vi "FipsAdjacent.vi"() -> (11 "Fips":i32[](array[numeric]))   [LabVIEW 2017] (continued)
\"Deuel County, NE\"\t31049\t\"Keith County, NE\"\t31101\n\"Deuel County, NE\"\t31049\t\"Perkins County, NE\"\t31135\n\"Dixon County, NE\"\t31051\t\"Cedar County, NE\"\t31027\n\"Dixon County, NE\"\t31051\t\"Dakota County, NE\"\t31043\n\"Dixon County, NE\"\t31051\t\"Dixon County, NE\"\t31051\n\"Dixon County, NE\"\t31051\t\"Thurston County, NE\"\t31173\n\"Dixon County, NE\"\t31051\t\"Wayne County, NE\"\t31179\n\"Dixon County, NE\"\t31051\t\"Clay County, SD\"\t46027\n\"Dixon County, NE\"\t31051\t\"Union County, SD\"\t46127\n\"Dodge County, NE\"\t31053\t\"Burt County, NE\"\t31021\n\"Dodge County, NE\"\t31053\t\"Butler County, NE\"\t31023\n\"Dodge County, NE\"\t31053\t\"Colfax County, NE\"\t31037\n\"Dodge County, NE\"\t31053\t\"Cuming County, NE\"\t31039\n\"Dodge County, NE\"\t31053\t\"Dodge County, NE\"\t31053\n\"Dodge County, NE\"\t31053\t\"Douglas County, NE\"\t31055\n\"Dodge County, NE\"\t31053\t\"Saunders County, NE\"\t31155\n\"Dodge County, NE\"\t31053\t\"Washington County, NE\"\t31177\n\"Douglas County, NE\"\t31055\t\"Pottawattamie County, IA\"\t19155\n\"Douglas County, NE\"\t31055\t\"Dodge County, NE\"\t31053\n\"Douglas County, NE\"\t31055\t\"Douglas County, NE\"\t31055\n\"Douglas County, NE\"\t31055\t\"Sarpy County, NE\"\t31153\n\"Douglas County, NE\"\t31055\t\"Saunders County, NE\"\t31155\n\"Douglas County, NE\"\t31055\t\"Washington County, NE\"\t31177\n\"Dundy County, NE\"\t31057\t\"Yuma County, CO\"\t08125\n\"Dundy County, NE\"\t31057\t\"Cheyenne County, KS\"\t20023\n\"Dundy County, NE\"\t31057\t\"Rawlins County, KS\"\t20153\n\"Dundy County, NE\"\t31057\t\"Chase County, NE\"\t31029\n\"Dundy County, NE\"\t31057\t\"Dundy County, NE\"\t31057\n\"Dundy County, NE\"\t31057\t\"Hayes County, NE\"\t31085\n\"Dundy County, NE\"\t31057\t\"Hitchcock County, NE\"\t31087\n\"Fillmore County, NE\"\t31059\t\"Clay County, NE\"\t31035\n\"Fillmore County, NE\"\t31059\t\"Fillmore County, NE\"\t31059\n\"Fillmore County, NE\"\t31059\t\"Jefferson County, NE\"\t31095\n\"Fillmore County, NE\"\t31059\t\"Nuckolls County, NE\"\t31129\n\"Fillmore County, NE\"\t31059\t\"Saline County, NE\"\t31151\n\"Fillmore County, NE\"\t31059\t\"Seward County, NE\"\t31159\n\"Fillmore County, NE\"\t31059\t\"Thayer County, NE\"\t31169\n\"Fillmore County, NE\"\t31059\t\"York County, NE\"\t31185\n\"Franklin County, NE\"\t31061\t\"Phillips County, KS\"\t20147\n\"Franklin County, NE\"\t31061\t\"Smith County, KS\"\t20183\n\"Franklin County, NE\"\t31061\t\"Franklin County, NE\"\t31061\n\"Franklin County, NE\"\t31061\t\"Harlan County, NE\"\t31083\n\"Franklin County, NE\"\t31061\t\"Kearney County, NE\"\t31099\n\"Franklin County, NE\"\t31061\t\"Phelps County, NE\"\t31137\n\"Franklin County, NE\"\t31061\t\"Webster County, NE\"\t31181\n\"Frontier County, NE\"\t31063\t\"Dawson County, NE\"\t31047\n\"Frontier County, NE\"\t31063\t\"Frontier County, NE\"\t31063\n\"Frontier County, NE\"\t31063\t\"Furnas County, NE\"\t31065\n\"Frontier County, NE\"\t31063\t\"Gosper County, NE\"\t31073\n\"Frontier County, NE\"\t31063\t\"Hayes County, NE\"\t31085\n\"Frontier County, NE\"\t31063\t\"Hitchcock County, NE\"\t31087\n\"Frontier County, NE\"\t31063\t\"Lincoln County, NE\"\t31111\n\"Frontier County, NE\"\t31063\t\"Red Willow County, NE\"\t31145\n\"Furnas County, NE\"\t31065\t\"Decatur County, KS\"\t20039\n\"Furnas County, NE\"\t31065\t\"Norton County, KS\"\t20137\n\"Furnas County, NE\"\t31065\t\"Frontier County, NE\"\t31063\n\"Furnas County, NE\"\t31065\t\"Furnas County, NE\"\t31065\n\"Furnas County, NE\"\t31065\t\"Gosper County, NE\"\t31073\n\"Furnas County, NE\"\t31065\t\"Harlan County, NE\"\t31083\n\"Furnas County, NE\"\t31065\t\"Phelps County, NE\"\t31137\n\"Furnas County, NE\"\t31065\t\"Red Willow County, NE\"\t31145\n\"Gage County, NE\"\t31067\t\"Marshall County, KS\"\t20117\n\"Gage County, NE\"\t31067\t\"Washington County, KS\"\t20201\n\"Gage County, NE\"\t31067\t\"Gage County, NE\"\t31067\n\"Gage County, NE\"\t31067\t\"Jefferson County, NE\"\t31095\n\"Gage County, NE\"\t31067\t\"Johnson County, NE\"\t31097\n\"Gage County, NE\"\t31067\t\"Lancaster County, NE\"\t31109\n\"Gage County, NE\"\t31067\t\"Otoe County, NE\"\t31131\n\"Gage County, NE\"\t31067\t\"Pawnee County, NE\"\t31133\n\"Gage County, NE\"\t31067\t\"Saline County, NE\"\t31151\n\"Garden County, NE\"\t31069\t\"Arthur County, NE\"\t31005\n\"Garden County, NE\"\t31069\t\"Cheyenne County, NE\"\t31033\n\"Garden County, NE\"\t31069\t\"Deuel County, NE\"\t31049\n\"Garden County, NE\"\t31069\t\"Garden County, NE\"\t31069\n\"Garden County, NE\"\t31069\t\"Grant County, NE\"\t31075\n\"Garden County, NE\"\t31069\t\"Keith County, NE\"\t31101\n\"Garden County, NE\"\t31069\t\"Morrill County, NE\"\t31123\n\"Garden County, NE\"\t31069\t\"Sheridan County, NE\"\t31161\n\"Garfield County, NE\"\t31071\t\"Custer County, NE\"\t31041\n\"Garfield County, NE\"\t31071\t\"Garfield County, NE\"\t31071\n\"Garfield County, NE\"\t31071\t\"Holt County, NE\"\t31089\n\"Garfield County, NE\"\t31071\t\"Loup County, NE\"\t31115\n\"Garfield County, NE\"\t31071\t\"Valley County, NE\"\t31175\n\"Garfield County, NE\"\t31071\t\"Wheeler County, NE\"\t31183\n\"Gosper County, NE\"\t31073\t\"Dawson County, NE\"\t31047\n\"Gosper County, NE\"\t31073\t\"Frontier County, NE\"\t31063\n\"Gosper County, NE\"\t31073\t\"Furnas County, NE\"\t31065\n\"Gosper County, NE\"\t31073\t\"Gosper County, NE\"\t31073\n\"Gosper County, NE\"\t31073\t\"Phelps County, NE\"\t31137\n\"Grant County, NE\"\t31075\t\"Arthur County, NE\"\t31005\n\"Grant County, NE\"\t31075\t\"Cherry County, NE\"\t31031\n\"Grant County, NE\"\t31075\t\"Garden County, NE\"\t31069\n\"Grant County, NE\"\t31075\t\"Grant County, NE\"\t31075\n\"Grant County, NE\"\t31075\t\"Hooker County, NE\"\t31091\n\"Grant County, NE\"\t31075\t\"Sheridan County, NE\"\t31161\n\"Greeley County, NE\"\t31077\t\"Boone County, NE\"\t31011\n\"Greeley County, NE\"\t31077\t\"Greeley County, NE\"\t31077\n\"Greeley County, NE\"\t31077\t\"Howard County, NE\"\t31093\n\"Greeley County, NE\"\t31077\t\"Nance County, NE\"\t31125\n\"Greeley County, NE\"\t31077\t\"Sherman County, NE\"\t31163\n\"Greeley County, NE\"\t31077\t\"Valley County, NE\"\t31175\n\"Greeley County, NE\"\t31077\t\"Wheeler County, NE\"\t31183\n\"Hall County, NE\"\t31079\t\"Adams County, NE\"\t31001\n\"Hall County, NE\"\t31079\t\"Buffalo County, NE\"\t31019\n\"Hall County, NE\"\t31079\t\"Hall County, NE\"\t31079\n\"Hall County, NE\"\t31079\t\"Hamilton County, NE\"\t31081\n\"Hall County, NE\"\t31079\t\"Howard County, NE\"\t31093\n\"Hall County, NE\"\t31079\t\"Merrick County, NE\"\t31121\n\"Hamilton County, NE\"\t31081\t\"Adams County, NE\"\t31001\n\"Hamilton County, NE\"\t31081\t\"Clay County, NE\"\t31035\n\"Hamilton County, NE\"\t31081\t\"Hall County, NE\"\t31079\n\"Hamilton County, NE\"\t31081\t\"Hamilton County, NE\"\t31081\n\"Hamilton County, NE\"\t31081\t\"Merrick County, NE\"\t31121\n\"Hamilton County, NE\"\t31081\t\"Polk County, NE\"\t31143\n\"Hamilton County, NE\"\t31081\t\"York County, NE\"\t31185\n\"Harlan County, NE\"\t31083\t\"Norton County, KS\"\t20137\n\"Harlan County, NE\"\t31083\t\"Phillips County, KS\"\t20147\n\"Harlan County, NE\"\t31083\t\"Franklin County, NE\"\t31061\n\"Harlan County, NE\"\t31083\t\"Furnas County, NE\"\t31065\n\"Harlan County, NE\"\t31083\t\"Harlan County, NE\"\t31083\n\"Harlan County, NE\"\t31083\t\"Kearney County, NE\"\t31099\n\"Harlan County, NE\"\t31083\t\"Phelps County, NE\"\t31137\n\"Hayes County, NE\"\t31085\t\"Chase County, NE\"\t31029\n\"Hayes County, NE\"\t31085\t\"Dundy County, NE\"\t31057\n\"Hayes County, NE\"\t31085\t\"Frontier County, NE\"\t31063\n\"Hayes County, NE\"\t31085\t\"Hayes County, NE\"\t31085\n\"Hayes County, NE\"\t31085\t\"Hitchcock County, NE\"\t31087\n\"Hayes County, NE\"\t31085\t\"Lincoln County, NE\"\t31111\n\"Hayes County, NE\"\t31085\t\"Perkins County, NE\"\t31135\n\"Hitchcock County, NE\"\t31087\t\"Rawlins County, KS\"\t20153\n\"Hitchcock County, NE\"\t31087\t\"Dundy County, NE\"\t31057\n\"Hitchcock County, NE\"\t31087\t\"Frontier County, NE\"\t31063\n\"Hitchcock County, NE\"\t31087\t\"Hayes County, NE\"\t31085\n\"Hitchcock County, NE\"\t31087\t\"Hitchcock County, NE\"\t31087\n\"Hitchcock County, NE\"\t31087\t\"Red Willow County, NE\"\t31145\n\"Holt County, NE\"\t31089\t\"Antelope County, NE\"\t31003\n\"Holt County, NE\"\t31089\t\"Boyd County, NE\"\t31015\n\"Holt County, NE\"\t31089\t\"Garfield County, NE\"\t31071\n\"Holt County, NE\"\t31089\t\"Holt County, NE\"\t31089\n\"Holt County, NE\"\t31089\t\"Keya Paha County, NE\"\t31103\n\"Holt County, NE\"\t31089\t\"Knox County, NE\"\t31107\n\"Holt County, NE\"\t31089\t\"Loup County, NE\"\t31115\n\"Holt County, NE\"\t31089\t\"Rock County, NE\"\t31149\n\"Holt County, NE\"\t31089\t\"Wheeler County, NE\"\t31183\n\"Hooker County, NE\"\t31091\t\"Arthur County, NE\"\t31005\n\"Hooker County, NE\"\t31091\t\"Cherry County, NE\"\t31031\n\"Hooker County, NE\"\t31091\t\"Grant County, NE\"\t31075\n\"Hooker County, NE\"\t31091\t\"Hooker County, NE\"\t31091\n\"Hooker County, NE\"\t31091\t\"McPherson County, NE\"\t31117\n\"Hooker County, NE\"\t31091\t\"Thomas County, NE\"\t31171\n\"Howard County, NE\"\t31093\t\"Buffalo County, NE\"\t31019\n\"Howard County, NE\"\t31093\t\"Greeley County, NE\"\t31077\n\"Howard County, NE\"\t31093\t\"Hall County, NE\"\t31079\n\"Howard County, NE\"\t31093\t\"Howard County, NE\"\t31093\n\"Howard County, NE\"\t31093\t\"Merrick County, NE\"\t31121\n\"Howard County, NE\"\t31093\t\"Nance County, NE\"\t31125\n\"Howard County, NE\"\t31093\t\"Sherman County, NE\"\t31163\n\"Jefferson County, NE\"\t31095\t\"Republic County, KS\"\t20157\n\"Jefferson County, NE\"\t31095\t\"Washington County, KS\"\t20201\n\"Jefferson County, NE\"\t31095\t\"Fillmore County, NE\"\t31059\n\"Jefferson County, NE\"\t31095\t\"Gage County, NE\"\t31067\n\"Jefferson County, NE\"\t31095\t\"Jefferson County, NE\"\t31095\n\"Jefferson County, NE\"\t31095\t\"Saline County, NE\"\t31151\n\"Jefferson County, NE\"\t31095\t\"Thayer County, NE\"\t31169\n\"Johnson County, NE\"\t31097\t\"Gage County, NE\"\t31067\n\"Johnson County, NE\"\t31097\t\"Johnson County, NE\"\t31097\n\"Johnson County, NE\"\t31097\t\"Lancaster County, NE\"\t31109\n\"Johnson County, NE\"\t31097\t\"Nemaha County, NE\"\t31127\n\"Johnson County, NE\"\t31097\t\"Otoe County, NE\"\t31131\n\"Johnson County, NE\"\t31097\t\"Pawnee County, NE\"\t31133\n\"Kearney County, NE\"\t31099\t\"Adams County, NE\"\t31001\n\"Kearney County, NE\"\t31099\t\"Buffalo County, NE\"\t31019\n\"Kearney County, NE\"\t31099\t\"Franklin County, NE\"\t31061\n\"Kearney County, NE\"\t31099\t\"Harlan County, NE\"\t31083\n\"Kearney County, NE\"\t31099\t\"Kearney County, NE\"\t31099\n\"Kearney County, NE\"\t31099\t\"Phelps County, NE\"\t31137\n\"Kearney County, NE\"\t31099\t\"Webster County, NE\"\t31181\n\"Keith County, NE\"\t31101\t\"Arthur County, NE\"\t31005\n\"Keith County, NE\"\t31101\t\"Deuel County, NE\"\t31049\n\"Keith County, NE\"\t31101\t\"Garden County, NE\"\t31069\n\"Keith County, NE\"\t31101\t\"Keith County, NE\"\t31101\n\"Keith County, NE\"\t31101\t\"Lincoln County, NE\"\t31111\n\"Keith County, NE\"\t31101\t\"McPherson County, NE\"\t31117\n\"Keith County, NE\"\t31101\t\"Perkins County, NE\"\t31135\n\"Keya Paha County, NE\"\t31103\t\"Boyd County, NE\"\t31015\n\"Keya Paha County, NE\"\t31103\t\"Brown County, NE\"\t31017\n\"Keya Paha County, NE\"\t31103\t\"Cherry County, NE\"\t31031\n\"Keya Paha County, NE\"\t31103\t\"Holt County, NE\"\t31089\n\"Keya Paha County, NE\"\t31103\t\"Keya Paha County, NE\"\t31103\n\"Keya Paha County, NE\"\t31103\t\"Rock County, NE\"\t31149\n\"Keya Paha County, NE\"\t31103\t\"Gregory County, SD\"\t46053\n\"Keya Paha County, NE\"\t31103\t\"Todd County, SD\"\t46121\n\"Keya Paha County, NE\"\t31103\t\"Tripp County, SD\"\t46123\n\"Kimball County, NE\"\t31105\t\"Logan County, CO\"\t08075\n\"Kimball County, NE\"\t31105\t\"Weld County, CO\"\t08123\n\"Kimball County, NE\"\t31105\t\"Banner County, NE\"\t31007\n\"Kimball County, NE\"\t31105\t\"Cheyenne County, NE\"\t31033\n\"Kimball County, NE\"\t31105\t\"Kimball County, NE\"\t31105\n\"Kimball County, NE\"\t31105\t\"Laramie County, WY\"\t56021\n\"Knox County, NE\"\t31107\t\"Antelope County, NE\"\t31003\n\"Knox County, NE\"\t31107\t\"Boyd County, NE\"\t31015\n\"Knox County, NE\"\t31107\t\"Cedar County, NE\"\t31027\n\"Knox County, NE\"\t31107\t\"Holt County, NE\"\t31089\n\"Knox County, NE\"\t31107\t\"Knox County, NE\"\t31107\n\"Knox County, NE\"\t31107\t\"Pierce County, NE\"\t31139\n\"Knox County, NE\"\t31107\t\"Bon Homme County, SD\"\t46009\n\"Knox County, NE\"\t31107\t\"Charles Mix County, SD\"\t46023\n\"Knox County, NE\"\t31107\t\"Yankton County, SD\"\t46135\n\"Lancaster County, NE\"\t31109\t\"Butler County, NE\"\t31023\n\"Lancaster County, NE\"\t31109\t\"Cass County, NE\"\t31025\n\"Lancaster County, NE\"\t31109\t\"Gage County, NE\"\t31067\n\"Lancaster County, NE\"\t31109\t\"Johnson County, NE\"\t31097\n\"Lancaster County, NE\"\t31109\t\"Lancaster County, NE\"\t31109\n\"Lancaster County, NE\"\t31109\t\"Otoe County, NE\"\t31131\n\"Lancaster County, NE\"\t31109\t\"Saline County, NE\"\t31151\n\"Lancaster County, NE\"\t31109\t\"Saunders County, NE\"\t31155\n\"Lancaster County, NE\"\t31109\t\"Seward County, NE\"\t31159\n\"Lincoln County, NE\"\t31111\t\"Custer County, NE\"\t31041\n\"Lincoln County, NE\"\t31111\t\"Dawson County, NE\"\t31047\n\"Lincoln County, NE\"\t31111\t\"Frontier County, NE\"\t31063\n\"Lincoln County, NE\"\t31111\t\"Hayes County, NE\"\t31085\n\"Lincoln County, NE\"\t31111\t\"Keith County, NE\"\t31101\n\"Lincoln County, NE\"\t31111\t\"Lincoln County, NE\"\t31111\n\"Lincoln County, NE\"\t31111\t\"Logan County, NE\"\t31113\n\"Lincoln County, NE\"\t31111\t\"McPherson County, NE\"\t31117\n\"Lincoln County, NE\"\t31111\t\"Perkins County, NE\"\t31135\n\"Logan County, NE\"\t31113\t\"Blaine County, NE\"\t31009\n\"Logan County, NE\"\t31113\t\"Custer County, NE\"\t31041\n\"Logan County, NE\"\t31113\t\"Lincoln County, NE\"\t31111\n\"Logan County, NE\"\t31113\t\"Logan County, NE\"\t31113\n\"Logan County, NE\"\t31113\t\"McPherson County, NE\"\t31117\n\"Logan County, NE\"\t31113\t\"Thomas County, NE\"\t31171\n\"Loup County, NE\"\t31115\t\"Blaine County, NE\"\t31009\n\"Loup County, NE\"\t31115\t\"Brown County, NE\"\t31017\n\"Loup County, NE\"\t31115\t\"Custer County, NE\"\t31041\n\"Loup County, NE\"\t31115\t\"Garfield County, NE\"\t31071\n\"Loup County, NE\"\t31115\t\"Holt County, NE\"\t31089\n\"Loup County, NE\"\t31115\t\"Loup County, NE\"\t31115\n\"Loup County, NE\"\t31115\t\"Rock County, NE\"\t31149\n\"McPherson County, NE\"\t31117\t\"Arthur County, NE\"\t31005\n\"McPherson County, NE\"\t31117\t\"Hooker County, NE\"\t31091\n\"McPherson County, NE\"\t31117\t\"Keith County, NE\"\t31101\n\"McPherson County, NE\"\t31117\t\"Lincoln County, NE\"\t31111\n\"McPherson County, NE\"\t31117\t\"Logan County, NE\"\t31113\n\"McPherson County, NE\"\t31117\t\"McPherson County, NE\"\t31117\n\"McPherson County, NE\"\t31117\t\"Thomas County, NE\"\t31171\n\"Madison County, NE\"\t31119\t\"Antelope County, NE\"\t31003\n\"Madison County, NE\"\t31119\t\"Boone County, NE\"\t31011\n\"Madison County, NE\"\t31119\t\"Madison County, NE\"\t31119\n\"Madison County, NE\"\t31119\t\"Pierce County, NE\"\t31139\n\"Madison County, NE\"\t31119\t\"Platte County, NE\"\t31141\n\"Madison County, NE\"\t31119\t\"Stanton County, NE\"\t31167\n\"Madison County, NE\"\t31119\t\"Wayne County, NE\"\t31179\n\"Merrick County, NE\"\t31121\t\"Hall County, NE\"\t31079\n\"Merrick County, NE\"\t31121\t\"Hamilton County, NE\"\t31081\n\"Merrick County, NE\"\t31121\t\"Howard County, NE\"\t31093\n\"Merrick County, NE\"\t31121\t\"Merrick County, NE\"\t31121\n\"Merrick County, NE\"\t31121\t\"Nance County, NE\"\t31125\n\"Merrick County, NE\"\t31121\t\"Platte County, NE\"\t31141\n\"Merrick County, NE\"\t31121\t\"Polk County, NE\"\t31143\n\"Morrill County, NE\"\t31123\t\"Banner County, NE\"\t31007\n\"Morrill County, NE\"\t31123\t\"Box Butte County, NE\"\t31013\n\"Morrill County, NE\"\t31123\t\"Cheyenne County, NE\"\t31033\n\"Morrill County, NE\"\t31123\t\"Garden County, NE\"\t31069\n\"Morrill County, NE\"\t31123\t\"Morrill County, NE\"\t31123\n\"Morrill County, NE\"\t31123\t\"Scotts Bluff County, NE\"\t31157\n\"Morrill County, NE\"\t31123\t\"Sheridan County, NE\"\t31161\n\"Nance County, NE\"\t31125\t\"Boone County, NE\"\t31011\n\"Nance County, NE\"\t31125\t\"Greeley County, NE\"\t31077\n\"Nance County, NE\"\t31125\t\"Howard County, NE\"\t31093\n\"Nance County, NE\"\t31125\t\"Merrick County, NE\"\t31121\n\"Nance County, NE\"\t31125\t\"Nance County, NE\"\t31125\n\"Nance County, NE\"\t31125\t\"Platte County, NE\"\t31141\n\"Nemaha County, NE\"\t31127\t\"Atchison County, MO\"\t29005\n\"Nemaha County, NE\"\t31127\t\"Holt County, MO\"\t29087\n\"Nemaha County, NE\"\t31127\t\"Johnson County, NE\"\t31097\n\"Nemaha County, NE\"\t31127\t\"Nemaha County, NE\"\t31127\n\"Nemaha County, NE\"\t31127\t\"Otoe County, NE\"\t31131\n\"Nemaha County, NE\"\t31127\t\"Pawnee County, NE\"\t31133\n\"Nemaha County, NE\"\t31127\t\"Richardson County, NE\"\t31147\n\"Nuckolls County, NE\"\t31129\t\"Jewell County, KS\"\t20089\n\"Nuckolls County, NE\"\t31129\t\"Republic County, KS\"\t20157\n\"Nuckolls County, NE\"\t31129\t\"Clay County, NE\"\t31035\n\"Nuckolls County, NE\"\t31129\t\"Fillmore County, NE\"\t31059\n\"Nuckolls County, NE\"\t31129\t\"Nuckolls County, NE\"\t31129\n\"Nuckolls County, NE\"\t31129\t\"Thayer County, NE\"\t31169\n\"Nuckolls County, NE\"\t31129\t\"Webster County, NE\"\t31181\n\"Otoe County, NE\"\t31131\t\"Fremont County, IA\"\t19071\n\"Otoe County, NE\"\t31131\t\"Atchison County, MO\"\t29005\n\"Otoe County, NE\"\t31131\t\"Cass County, NE\"\t31025\n\"Otoe County, NE\"\t31131\t\"Gage County, NE\"\t31067\n\"Otoe County, NE\"\t31131\t\"Johnson County, NE\"\t31097\n\"Otoe County, NE\"\t31131\t\"Lancaster County, NE\"\t31109\n\"Otoe County, NE\"\t31131\t\"Nemaha County, NE\"\t31127\n\"Otoe County, NE\"\t31131\t\"Otoe County, NE\"\t31131\n\"Pawnee County, NE\"\t31133\t\"Marshall County, KS\"\t20117\n\"Pawnee County, NE\"\t31133\t\"Nemaha County, KS\"\t20131\n\"Pawnee County, NE\"\t31133\t\"Gage County, NE\"\t31067\n\"Pawnee County, NE\"\t31133\t\"Johnson County, NE\"\t31097\n\"Pawnee County, NE\"\t31133\t\"Nemaha County, NE\"\t31127\n\"Pawnee County, NE\"\t31133\t\"Pawnee County, NE\"\t31133\n\"Pawnee County, NE\"\t31133\t\"Richardson County, NE\"\t31147\n\"Perkins County, NE\"\t31135\t\"Phillips County, CO\"\t08095\n\"Perkins County, NE\"\t31135\t\"Sedgwick County, CO\"\t08115\n\"Perkins County, NE\"\t31135\t\"Chase County, NE\"\t31029\n\"Perkins County, NE\"\t31135\t\"Deuel County, NE\"\t31049\n\"Perkins County, NE\"\t31135\t\"Hayes County, NE\"\t31085\n\"Perkins County, NE\"\t31135\t\"Keith County, NE\"\t31101\n\"Perkins County, NE\"\t31135\t\"Lincoln County, NE\"\t31111\n\"Perkins County, NE\"\t31135\t\"Perkins County, NE\"\t31135\n\"Phelps County, NE\"\t31137\t\"Buffalo County, NE\"\t31019\n\"Phelps County, NE\"\t31137\t\"Dawson County, NE\"\t31047\n\"Phelps County, NE\"\t31137\t\"Franklin County, NE\"\t31061\n\"Phelps County, NE\"\t31137\t\"Furnas County, NE\"\t31065\n\"Phelps County, NE\"\t31137\t\"Gosper County, NE\"\t31073\n\"Phelps County, NE\"\t31137\t\"Harlan County, NE\"\t31083\n\"Phelps County, NE\"\t31137\t\"Kearney County, NE\"\t31099\n\"Phelps County, NE\"\t31137\t\"Phelps County, NE\"\t31137\n\"Pierce County, NE\"\t31139\t\"Antelope County, NE\"\t31003\n\"Pierce County, NE\"\t31139\t\"Cedar County, NE\"\t31027\n\"Pierce County, NE\"\t31139\t\"Knox County, NE\"\t31107\n\"Pierce County, NE\"\t31139\t\"Madison County, NE\"\t31119\n\"Pierce County, NE\"\t31139\t\"Pierce County, NE\"\t31139\n\"Pierce County, NE\"\t31139\t\"Stanton County, NE\"\t31167\n\"Pierce County, NE\"\t31139\t\"Wayne County, NE\"\t31179\n\"Platte County, NE\"\t31141\t\"Boone County, NE\"\t31011\n\"Platte County, NE\"\t31141\t\"Butler County, NE\"\t31023\n\"Platte County, NE\"\t31141\t\"Colfax County, NE\"\t31037\n\"Platte County, NE\"\t31141\t\"Madison County, NE\"\t31119\n\"Platte County, NE\"\t31141\t\"Merrick County, NE\"\t31121\n\"Platte County, NE\"\t31141\t\"Nance County, NE\"\t31125\n\"Platte County, NE\"\t31141\t\"Platte County, NE\"\t31141\n\"Platte County, NE\"\t31141\t\"Polk County, NE\"\t31143\n\"Platte County, NE\"\t31141\t\"Stanton County, NE\"\t31167\n\"Polk County, NE\"\t31143\t\"Butler County, NE\"\t31023\n\"Polk County, NE\"\t31143\t\"Hamilton County, NE\"\t31081\n\"Polk County, NE\"\t31143\t\"Merrick County, NE\"\t31121\n\"Polk County, NE\"\t31143\t\"Platte County, NE\"\t31141\n\"Polk County, NE\"\t31143\t\"Polk County, NE\"\t31143\n\"Polk County, NE\"\t31143\t\"Seward County, NE\"\t31159\n\"Polk County, NE\"\t31143\t\"York County, NE\"\t31185\n\"Red Willow County, NE\"\t31145\t\"Decatur County, KS\"\t20039\n\"Red Willow County, NE\"\t31145\t\"Rawlins County, KS\"\t20153\n\"Red Willow County, NE\"\t31145\t\"Frontier County, NE\"\t31063\n\"Red Willow County, NE\"\t31145\t\"Furnas County, NE\"\t31065\n\"Red Willow County, NE\"\t31145\t\"Hitchcock County, NE\"\t31087\n\"Red Willow County, NE\"\t31145\t\"Red Willow County, NE\"\t31145\n\"Richardson County, NE\"\t31147\t\"Brown County, KS\"\t20013\n\"Richardson County, NE\"\t31147\t\"Doniphan County, KS\"\t20043\n\"Richardson County, NE\"\t31147\t\"Nemaha County, KS\"\t20131\n\"Richardson County, NE\"\t31147\t\"Holt County, MO\"\t29087\n\"Richardson County, NE\"\t31147\t\"Nemaha County, NE\"\t31127\n\"Richardson County, NE\"\t31147\t\"Pawnee County, NE\"\t31133\n\"Richardson County, NE\"\t31147\t\"Richardson County, NE\"\t31147\n\"Rock County, NE\"\t31149\t\"Boyd County, NE\"\t31015\n\"Rock County, NE\"\t31149\t\"Brown County, NE\"\t31017\n\"Rock County, NE\"\t31149\t\"Holt County, NE\"\t31089\n\"Rock County, NE\"\t31149\t\"Keya Paha County, NE\"\t31103\n\"Rock County, NE\"\t31149\t\"Loup County, NE\"\t31115\n\"Rock County, NE\"\t31149\t\"Rock County, NE\"\t31149\n\"Saline County, NE\"\t31151\t\"Fillmore County, NE\"\t31059\n\"Saline County, NE\"\t31151\t\"Gage County, NE\"\t31067\n\"Saline County, NE\"\t31151\t\"Jefferson County, NE\"\t31095\n\"Saline County, NE\"\t31151\t\"Lancaster County, NE\"\t31109\n\"Saline County, NE\"\t31151\t\"Saline County, NE\"\t31151\n\"Saline County, NE\"\t31151\t\"Seward County, NE\"\t31159\n\"Saline County, NE\"\t31151\t\"Thayer County, NE\"\t31169\n\"Saline County, NE\"\t31151\t\"York County, NE\"\t31185\n\"Sarpy County, NE\"\t31153\t\"Mills County, IA\"\t19129\n\"Sarpy County, NE\"\t31153\t\"Pottawattamie County, IA\"\t19155\n\"Sarpy County, NE\"\t31153\t\"Cass County, NE\"\t31025\n\"Sarpy County, NE\"\t31153\t\"Douglas County, NE\"\t31055\n\"Sarpy County, NE\"\t31153\t\"Sarpy County, NE\"\t31153\n\"Sarpy County, NE\"\t31153\t\"Saunders County, NE\"\t31155\n\"Saunders County, NE\"\t31155\t\"Butler County, NE\"\t31023\n\"Saunders County, NE\"\t31155\t\"Cass County, NE\"\t31025\n\"Saunders County, NE\"\t31155\t\"Dodge County, NE\"\t31053\n\"Saunders County, NE\"\t31155\t\"Douglas County, NE\"\t31055\n\"Saunders County, NE\"\t31155\t\"Lancaster County, NE\"\t31109\n\"Saunders County, NE\"\t31155\t\"Sarpy County, NE\"\t31153\n\"Saunders County, NE\"\t31155\t\"Saunders County, NE\"\t31155\n\"Scotts Bluff County, NE\"\t31157\t\"Banner County, NE\"\t31007\n\"Scotts Bluff County, NE\"\t31157\t\"Box Butte County, NE\"\t31013\n\"Scotts Bluff County, NE\"\t31157\t\"Morrill County, NE\"\t31123\n\"Scotts Bluff County, NE\"\t31157\t\"Scotts Bluff County, NE\"\t31157\n\"Scotts Bluff County, NE\"\t31157\t\"Sioux County, NE\"\t31165\n\"Scotts Bluff County, NE\"\t31157\t\"Goshen County, WY\"\t56015\n\"Seward County, NE\"\t31159\t\"Butler County, NE\"\t31023\n\"Seward County, NE\"\t31159\t\"Fillmore County, NE\"\t31059\n\"Seward County, NE\"\t31159\t\"Lancaster County, NE\"\t31109\n\"Seward County, NE\"\t31159\t\"Polk County, NE\"\t31143\n\"Seward County, NE\"\t31159\t\"Saline County, NE\"\t31151\n\"Seward County, NE\"\t31159\t\"Seward County, NE\"\t31159\n\"Seward County, NE\"\t31159\t\"York County, NE\"\t31185\n\"Sheridan County, NE\"\t31161\t\"Box Butte County, NE\"\t31013\n\"Sheridan County, NE\"\t31161\t\"Cherry County, NE\"\t31031\n\"Sheridan County, NE\"\t31161\t\"Dawes County, NE\"\t31045\n\"Sheridan County, NE\"\t31161\t\"Garden County, NE\"\t31069\n\"Sheridan County, NE\"\t31161\t\"Grant County, NE\"\t31075\n\"Sheridan County, NE\"\t31161\t\"Morrill County, NE\"\t31123\n\"Sheridan County, NE\"\t31161\t\"Sheridan County, NE\"\t31161\n\"Sheridan County, NE\"\t31161\t\"Shannon County, SD\"\t46113\n\"Sherman County, NE\"\t31163\t\"Buffalo County, NE\"\t31019\n\"Sherman County, NE\"\t31163\t\"Custer County, NE\"\t31041\n\"Sherman County, NE\"\t31163\t\"Greeley County, NE\"\t31077\n\"Sherman County, NE\"\t31163\t\"Howard County, NE\"\t31093\n\"Sherman County, NE\"\t31163\t\"Sherman County, NE\"\t31163\n\"Sherman County, NE\"\t31163\t\"Valley County, NE\"\t31175\n\"Sioux County, NE\"\t31165\t\"Box Butte County, NE\"\t31013\n\"Sioux County, NE\"\t31165\t\"Dawes County, NE\"\t31045\n\"Sioux County, NE\"\t31165\t\"Scotts Bluff County, NE\"\t31157\n\"Sioux County, NE\"\t31165\t\"Sioux County, NE\"\t31165\n\"Sioux County, NE\"\t31165\t\"Fall River County, SD\"\t46047\n\"Sioux County, NE\"\t31165\t\"Goshen County, WY\"\t56015\n\"Sioux County, NE\"\t31165\t\"Niobrara County, WY\"\t56027\n\"Stanton County, NE\"\t31167\t\"Colfax County, NE\"\t31037\n\"Stanton County, NE\"\t31167\t\"Cuming County, NE\"\t31039\n\"Stanton County, NE\"\t31167\t\"Madison County, NE\"\t31119\n\"Stanton County, NE\"\t31167\t\"Pierce County, NE\"\t31139\n\"Stanton County, NE\"\t31167\t\"Platte County, NE\"\t31141\n\"Stanton County, NE\"\t31167\t\"Stanton County, NE\"\t31167\n\"Stanton County, NE\"\t31167\t\"Wayne County, NE\"\t31179\n\"Thayer County, NE\"\t31169\t\"Republic County, KS\"\t20157\n\"Thayer County, NE\"\t31169\t\"Washington County, KS\"\t20201\n\"Thayer County, NE\"\t31169\t\"Fillmore County, NE\"\t31059\n\"Thayer County, NE\"\t31169\t\"Jefferson County, NE\"\t31095\n\"Thayer County, NE\"\t31169\t\"Nuckolls County, NE\"\t31129\n\"Thayer County, NE\"\t31169\t\"Saline County, NE\"\t31151\n\"Thayer County, NE\"\t31169\t\"Thayer County, NE\"\t31169\n\"Thomas County, NE\"\t31171\t\"Blaine County, NE\"\t31009\n\"Thomas County, NE\"\t31171\t\"Cherry County, NE\"\t31031\n\"Thomas County, NE\"\t31171\t\"Hooker County, NE\"\t31091\n\"Thomas County, NE\"\t31171\t\"Logan County, NE\"\t31113\n\"Thomas County, NE\"\t31171\t\"McPherson County, NE\"\t31117\n\"Thomas County, NE\"\t31171\t\"Thomas County, NE\"\t31171\n\"Thurston County, NE\"\t31173\t\"Monona County, IA\"\t19133\n\"Thurston County, NE\"\t31173\t\"Woodbury County, IA\"\t19193\n\"Thurston County, NE\"\t31173\t\"Burt County, NE\"\t31021\n\"Thurston County, NE\"\t31173\t\"Cuming County, NE\"\t31039\n\"Thurston County, NE\"\t31173\t\"Dakota County, NE\"\t31043\n\"Thurston County, NE\"\t31173\t\"Dixon County, NE\"\t31051\n\"Thurston County, NE\"\t31173\t\"Thurston County, NE\"\t31173\n\"Thurston County, NE\"\t31173\t\"Wayne County, NE\"\t31179\n\"Valley County, NE\"\t31175\t\"Custer County, NE\"\t31041\n\"Valley County, NE\"\t31175\t\"Garfield County, NE\"\t31071\n\"Valley County, NE\"\t31175\t\"Greeley County, NE\"\t31077\n\"Valley County, NE\"\t31175\t\"Sherman County, NE\"\t31163\n\"Valley County, NE\"\t31175\t\"Valley County, NE\"\t31175\n\"Valley County, NE\"\t31175\t\"Wheeler County, NE\"\t31183\n\"Washington County, NE\"\t31177\t\"Harrison County, IA\"\t19085\n\"Washington County, NE\"\t31177\t\"Pottawattamie County, IA\"\t19155\n\"Washington County, NE\"\t31177\t\"Burt County, NE\"\t31021\n\"Washington County, NE\"\t31177\t\"Dodge County, NE\"\t31053\n\"Washington County, NE\"\t31177\t\"Douglas County, NE\"\t31055\n\"Washington County, NE\"\t31177\t\"Washington County, NE\"\t31177\n\"Wayne County, NE\"\t31179\t\"Cedar County, NE\"\t31027\n\"Wayne County, NE\"\t31179\t\"Cuming County, NE\"\t31039\n\"Wayne County, NE\"\t31179\t\"Dixon County, NE\"\t31051\n\"Wayne County, NE\"\t31179\t\"Madison County, NE\"\t31119\n\"Wayne County, NE\"\t31179\t\"Pierce County, NE\"\t31139\n\"Wayne County, NE\"\t31179\t\"Stanton County, NE\"\t31167\n\"Wayne County, NE\"\t31179\t\"Thurston County, NE\"\t31173\n\"Wayne County, NE\"\t31179\t\"Wayne County, NE\"\t31179\n\"Webster County, NE\"\t31181\t\"Jewell County, KS\"\t20089\n\"Webster County, NE\"\t31181\t\"Smith County, KS\"\t20183\n\"Webster County, NE\"\t31181\t\"Adams County, NE\"\t31001\n\"Webster County, NE\"\t31181\t\"Clay County, NE\"\t31035\n\"Webster County, NE\"\t31181\t\"Franklin County, NE\"\t31061\n\"Webster County, NE\"\t31181\t\"Kearney County, NE\"\t31099\n\"Webster County, NE\"\t31181\t\"Nuckolls County, NE\"\t31129\n\"Webster County, NE\"\t31181\t\"Webster County, NE\"\t31181\n\"Wheeler County, NE\"\t31183\t\"Antelope County, NE\"\t31003\n\"Wheeler County, NE\"\t31183\t\"Boone County, NE\"\t31011\n\"Wheeler County, NE\"\t31183\t\"Garfield County, NE\"\t31071\n\"Wheeler County, NE\"\t31183\t\"Greeley County, NE\"\t31077\n\"Wheeler County, NE\"\t31183\t\"Holt County, NE\"\t31089\n\"Wheeler County, NE\"\t31183\t\"Valley County, NE\"\t31175\n\"Wheeler County, NE\"\t31183\t\"Wheeler County, NE\"\t31183\n\"York County, NE\"\t31185\t\"Butler County, NE\"\t31023\n\"York County, NE\"\t31185\t\"Clay County, NE\"\t31035\n\"York County, NE\"\t31185\t\"Fillmore County, NE\"\t31059\n\"York County, NE\"\t31185\t\"Hamilton County, NE\"\t31081\n\"York County, NE\"\t31185\t\"Polk County, NE\"\t31143\n\"York County, NE\"\t31185\t\"Saline County, NE\"\t31151\n\"York County, NE\"\t31185\t\"Seward County, NE\"\t31159\n\"York County, NE\"\t31185\t\"York County, NE\"\t31185\n\"Churchill County, NV\"\t32001\t\"Churchill County, NV\"\t32001\n\"Churchill County, NV\"\t32001\t\"Lander County, NV\"\t32015\n\"Churchill County, NV\"\t32001\t\"Lyon County, NV\"\t32019\n\"Churchill County, NV\"\t32001\t\"Mineral County, NV\"\t32021\n\"Churchill County, NV\"\t32001\t\"Nye County, NV\"\t32023\n\"Churchill County, NV\"\t32001\t\"Pershing County, NV\"\t32027\n\"Churchill County, NV\"\t32001\t\"Washoe County, NV\"\t32031\n\"Clark County, NV\"\t32003\t\"Mohave County, AZ\"\t04015\n\"Clark County, NV\"\t32003\t\"Inyo County, CA\"\t06027\n\"Clark County, NV\"\t32003\t\"San Bernardino County, CA\"\t06071\n\"Clark County, NV\"\t32003\t\"Clark County, NV\"\t32003\n\"Clark County, NV\"\t32003\t\"Lincoln County, NV\"\t32017\n\"Clark County, NV\"\t32003\t\"Nye County, NV\"\t32023\n\"Douglas County, NV\"\t32005\t\"Alpine County, CA\"\t06003\n\"Douglas County, NV\"\t32005\t\"El Dorado County, CA\"\t06017\n\"Douglas County, NV\"\t32005\t\"Mono County, CA\"\t06051\n\"Douglas County, NV\"\t32005\t\"Placer County, CA\"\t06061\n\"Douglas County, NV\"\t32005\t\"Douglas County, NV\"\t32005\n\"Douglas County, NV\"\t32005\t\"Lyon County, NV\"\t32019\n\"Douglas County, NV\"\t32005\t\"Carson City, NV\"\t32510\n\"Elko County, NV\"\t32007\t\"Cassia County, ID\"\t16031\n\"Elko County, NV\"\t32007\t\"Owyhee County, ID\"\t16073\n\"Elko County, NV\"\t32007\t\"Twin Falls County, ID\"\t16083\n\"Elko County, NV\"\t32007\t\"Elko County, NV\"\t32007\n\"Elko County, NV\"\t32007\t\"Eureka County, NV\"\t32011\n\"Elko County, NV\"\t32007\t\"Humboldt County, NV\"\t32013\n\"Elko County, NV\"\t32007\t\"Lander County, NV\"\t32015\n\"Elko County, NV\"\t32007\t\"White Pine County, NV\"\t32033\n\"Elko County, NV\"\t32007\t\"Box Elder County, UT\"\t49003\n\"Elko County, NV\"\t32007\t\"Tooele County, UT\"\t49045\n\"Esmeralda County, NV\"\t32009\t\"Inyo County, CA\"\t06027\n\"Esmeralda County, NV\"\t32009\t\"Mono County, CA\"\t06051\n\"Esmeralda County, NV\"\t32009\t\"Esmeralda County, NV\"\t32009\n\"Esmeralda County, NV\"\t32009\t\"Mineral County, NV\"\t32021\n\"Esmeralda County, NV\"\t32009\t\"Nye County, NV\"\t32023\n\"Eureka County, NV\"\t32011\t\"Elko County, NV\"\t32007\n\"Eureka County, NV\"\t32011\t\"Eureka County, NV\"\t32011\n\"Eureka County, NV\"\t32011\t\"Lander County, NV\"\t32015\n\"Eureka County, NV\"\t32011\t\"Nye County, NV\"\t32023\n\"Eureka County, NV\"\t32011\t\"White Pine County, NV\"\t32033\n\"Humboldt County, NV\"\t32013\t\"Owyhee County, ID\"\t16073\n\"Humboldt County, NV\"\t32013\t\"Elko County, NV\"\t32007\n\"Humboldt County, NV\"\t32013\t\"Humboldt County, NV\"\t32013\n\"Humboldt County, NV\"\t32013\t\"Lander County, NV\"\t32015\n\"Humboldt County, NV\"\t32013\t\"Pershing County, NV\"\t32027\n\"Humboldt County, NV\"\t32013\t\"Washoe County, NV\"\t32031\n\"Humboldt County, NV\"\t32013\t\"Harney County, OR\"\t41025\n\"Humboldt County, NV\"\t32013\t\"Malheur County, OR\"\t41045\n\"Lander County, NV\"\t32015\t\"Churchill County, NV\"\t32001\n\"Lander County, NV\"\t32015\t\"Elko County, NV\"\t32007\n\"Lander County, NV\"\t32015\t\"Eureka County, NV\"\t32011\n\"Lander County, NV\"\t32015\t\"Humboldt County, NV\"\t32013\n\"Lander County, NV\"\t32015\t\"Lander County, NV\"\t32015\n\"Lander County, NV\"\t32015\t\"Nye County, NV\"\t32023\n\"Lander County, NV\"\t32015\t\"Pershing County, NV\"\t32027\n\"Lincoln County, NV\"\t32017\t\"Mohave County, AZ\"\t04015\n\"Lincoln County, NV\"\t32017\t\"Clark County, NV\"\t32003\n\"Lincoln County, NV\"\t32017\t\"Lincoln County, NV\"\t32017\n\"Lincoln County, NV\"\t32017\t\"Nye County, NV\"\t32023\n\"Lincoln County, NV\"\t32017\t\"White Pine County, NV\"\t32033\n\"Lincoln County, NV\"\t32017\t\"Beaver County, UT\"\t49001\n\"Lincoln County, NV\"\t32017\t\"Iron County, UT\"\t49021\n\"Lincoln County, NV\"\t32017\t\"Millard County, UT\"\t49027\n\"Lincoln County, NV\"\t32017\t\"Washington County, UT\"\t49053\n\"Lyon County, NV\"\t32019\t\"Mono County, CA\"\t06051\n\"Lyon County, NV\"\t32019\t\"Churchill County, NV\"\t32001\n\"Lyon County, NV\"\t32019\t\"Douglas County, NV\"\t32005\n\"Lyon County, NV\"\t32019\t\"Lyon County, NV\"\t32019\n\"Lyon County, NV\"\t32019\t\"Mineral County, NV\"\t32021\n\"Lyon County, NV\"\t32019\t\"Storey County, NV\"\t32029\n\"Lyon County, NV\"\t32019\t\"Washoe County, NV\"\t32031\n\"Lyon County, NV\"\t32019\t\"Carson City, NV\"\t32510\n\"Mineral County, NV\"\t32021\t\"Mono County, CA\"\t06051\n\"Mineral County, NV\"\t32021\t\"Churchill County, NV\"\t32001\n\"Mineral County, NV\"\t32021\t\"Esmeralda County, NV\"\t32009\n\"Mineral County, NV\"\t32021\t\"Lyon County, NV\"\t32019\n\"Mineral County, NV\"\t32021\t\"Mineral County, NV\"\t32021\n\"Mineral County, NV\"\t32021\t\"Nye County, NV\"\t32023\n\"Nye County, NV\"\t32023\t\"Inyo County, CA\"\t06027\n\"Nye County, NV\"\t32023\t\"Churchill County, NV\"\t32001\n\"Nye County, NV\"\t32023\t\"Clark County, NV\"\t32003\n\"Nye County, NV\"\t32023\t\"Esmeralda County, NV\"\t32009\n\"Nye County, NV\"\t32023\t\"Eureka County, NV\"\t32011\n\"Nye County, NV\"\t32023\t\"Lander County, NV\"\t32015\n\"Nye County, NV\"\t32023\t\"Lincoln County, NV\"\t32017\n\"Nye County, NV\"\t32023\t\"Mineral County, NV\"\t32021\n\"Nye County, NV\"\t32023\t\"Nye County, NV\"\t32023\n\"Nye County, NV\"\t32023\t\"White Pine County, NV\"\t32033\n\"Pershing County, NV\"\t32027\t\"Churchill County, NV\"\t32001\n\"Pershing County, NV\"\t32027\t\"Humboldt County, NV\"\t32013\n\"Pershing County, NV\"\t32027\t\"Lander County, NV\"\t32015\n\"Pershing County, NV\"\t32027\t\"Pershing County, NV\"\t32027\n\"Pershing County, NV\"\t32027\t\"Washoe County, NV\"\t32031\n\"Storey County, NV\"\t32029\t\"Lyon County, NV\"\t32019\n\"Storey County, NV\"\t32029\t\"Storey County, NV\"\t32029\n\"Storey County, NV\"\t32029\t\"Washoe County, NV\"\t32031\n\"Storey County, NV\"\t32029\t\"Carson City, NV\"\t32510\n\"Washoe County, NV\"\t32031\t\"Lassen County, CA\"\t06035\n\"Washoe County, NV\"\t32031\t\"Modoc County, CA\"\t06049\n\"Washoe County, NV\"\t32031\t\"Nevada County, CA\"\t06057\n\"Washoe County, NV\"\t32031\t\"Placer County, CA\"\t06061\n\"Washoe County, NV\"\t32031\t\"Sierra County, CA\"\t06091\n\"Washoe County, NV\"\t32031\t\"Churchill County, NV\"\t32001\n\"Washoe County, NV\"\t32031\t\"Humboldt County, NV\"\t32013\n\"Washoe County, NV\"\t32031\t\"Lyon County, NV\"\t32019\n\"Washoe County, NV\"\t32031\t\"Pershing County, NV\"\t32027\n\"Washoe County, NV\"\t32031\t\"Storey County, NV\"\t32029\n\"Washoe County, NV\"\t32031\t\"Washoe County, NV\"\t32031\n\"Washoe County, NV\"\t32031\t\"Carson City, NV\"\t32510\n\"Washoe County, NV\"\t32031\t\"Harney County, OR\"\t41025\n\"Washoe County, NV\"\t32031\t\"Lake County, OR\"\t41037\n\"White Pine County, NV\"\t32033\t\"Elko County, NV\"\t32007\n\"White Pine County, NV\"\t32033\t\"Eureka County, NV\"\t32011\n\"White Pine County, NV\"\t32033\t\"Lincoln County, NV\"\t32017\n\"White Pine County, NV\"\t32033\t\"Nye County, NV\"\t32023\n\"White Pine County, NV\"\t32033\t\"White Pine County, NV\"\t32033\n\"White Pine County, NV\"\t32033\t\"Juab County, UT\"\t49023\n\"White Pine County, NV\"\t32033\t\"Millard County, UT\"\t49027\n\"White Pine County, NV\"\t32033\t\"Tooele County, UT\"\t49045\n\"Carson City, NV\"\t32510\t\"Placer County, CA\"\t06061\n\"Carson City, NV\"\t32510\t\"Douglas County, NV\"\t32005\n\"Carson City, NV\"\t32510\t\"Lyon County, NV\"\t32019\n\"Carson City, NV\"\t32510\t\"Storey County, NV\"\t32029\n\"Carson City, NV\"\t32510\t\"Washoe County, NV\"\t32031\n\"Carson City, NV\"\t32510\t\"Carson City, NV\"\t32510\n\"Belknap County, NH\"\t33001\t\"Belknap County, NH\"\t33001\n\"Belknap County, NH\"\t33001\t\"Carroll County, NH\"\t33003\n\"Belknap County, NH\"\t33001\t\"Grafton County, NH\"\t33009\n\"Belknap County, NH\"\t33001\t\"Merrimack County, NH\"\t33013\n\"Belknap County, NH\"\t33001\t\"Strafford County, NH\"\t33017\n\"Carroll County, NH\"\t33003\t\"Oxford County, ME\"\t23017\n\"Carroll County, NH\"\t33003\t\"York County, ME\"\t23031\n\"Carroll County, NH\"\t33003\t\"Belknap County, NH\"\t33001\n\"Carroll County, NH\"\t33003\t\"Carroll County, NH\"\t33003\n\"Carroll County, NH\"\t33003\t\"Coos County, NH\"\t33007\n\"Carroll County, NH\"\t33003\t\"Grafton County, NH\"\t33009\n\"Carroll County, NH\"\t33003\t\"Strafford County, NH\"\t33017\n\"Cheshire County, NH\"\t33005\t\"Franklin County, MA\"\t25011\n\"Cheshire County, NH\"\t33005\t\"Worcester County, MA\"\t25027\n\"Cheshire County, NH\"\t33005\t\"Cheshire County, NH\"\t33005\n\"Cheshire County, NH\"\t33005\t\"Hillsborough County, NH\"\t33011\n\"Cheshire County, NH\"\t33005\t\"Sullivan County, NH\"\t33019\n\"Cheshire County, NH\"\t33005\t\"Windham County, VT\"\t50025\n\"Coos County, NH\"\t33007\t\"Oxford County, ME\"\t23017\n\"Coos County, NH\"\t33007\t\"Carroll County, NH\"\t33003\n\"Coos County, NH\"\t33007\t\"Coos County, NH\"\t33007\n\"Coos County, NH\"\t33007\t\"Grafton County, NH\"\t33009\n\"Coos County, NH\"\t33007\t\"Essex County, VT\"\t50009\n\"Grafton County, NH\"\t33009\t\"Belknap County, NH\"\t33001\n\"Grafton County, NH\"\t33009\t\"Carroll County, NH\"\t33003\n\"Grafton County, NH\"\t33009\t\"Coos County, NH\"\t33007\n\"Grafton County, NH\"\t33009\t\"Grafton County, NH\"\t33009\n\"Grafton County, NH\"\t33009\t\"Merrimack County, NH\"\t33013\n\"Grafton County, NH\"\t33009\t\"Sullivan County, NH\"\t33019\n\"Grafton County, NH\"\t33009\t\"Caledonia County, VT\"\t50005\n\"Grafton County, NH\"\t33009\t\"Essex County, VT\"\t50009\n\"Grafton County, NH\"\t33009\t\"Orange County, VT\"\t50017\n\"Grafton County, NH\"\t33009\t\"Windsor County, VT\"\t50027\n\"Hillsborough County, NH\"\t33011\t\"Essex County, MA\"\t25009\n\"Hillsborough County, NH\"\t33011\t\"Middlesex County, MA\"\t25017\n\"Hillsborough County, NH\"\t33011\t\"Worcester County, MA\"\t25027\n\"Hillsborough County, NH\"\t33011\t\"Cheshire County, NH\"\t33005\n\"Hillsborough County, NH\"\t33011\t\"Hillsborough County, NH\"\t33011\n\"Hillsborough County, NH\"\t33011\t\"Merrimack County, NH\"\t33013\n\"Hillsborough County, NH\"\t33011\t\"Rockingham County, NH\"\t33015\n\"Hillsborough County, NH\"\t33011\t\"Sullivan County, NH\"\t33019\n\"Merrimack County, NH\"\t33013\t\"Belknap County, NH\"\t33001\n\"Merrimack County, NH\"\t33013\t\"Grafton County, NH\"\t33009\n\"Merrimack County, NH\"\t33013\t\"Hillsborough County, NH\"\t33011\n\"Merrimack County, NH\"\t33013\t\"Merrimack County, NH\"
